vi "3_Extract Numbers_solution.vi"(11 "String":string="yi 2 -3 4.0 5.5") -> (3 "Result: Extracted Numbers":dbl[](array[numeric]) format="%#.6g")   [LabVIEW 2014]
panel:
  # "Extract Numbers from string and display in an array.\nThis picture is an example"
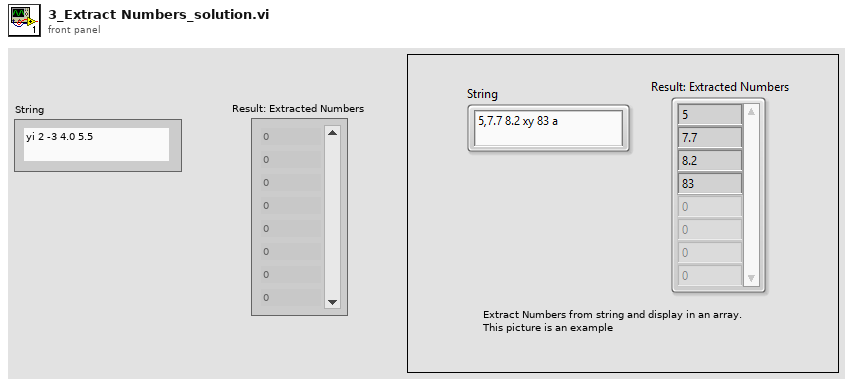
[diagram p1: front panel]
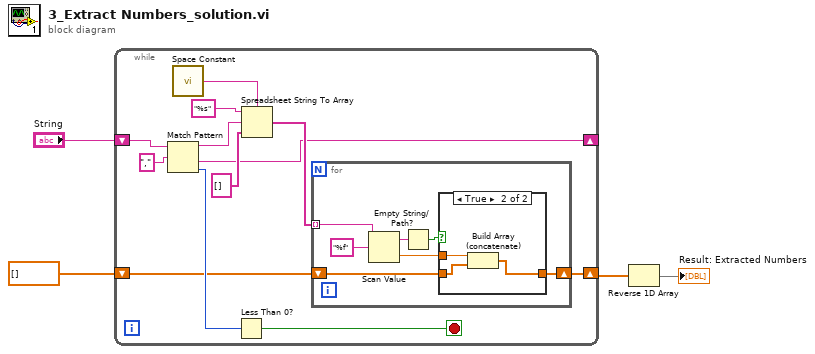
[diagram p0: block diagram]
diagram:
  n1 = while {
    shift-right: [w6] -> _
    shift-left: "String" -> [w16]
    shift-right: [w9] -> w2
    shift-left: dbl[] [] -> [w10]
    stop <- w13 stop-if-true
    n2 = Match Pattern(string=w16, regular expression=",") -> (before substring=w7:string, after substring=w6:string, offset past match=w14:i32)  [unwired: 1 in, 1 out]
    n3 = call <vilib>:"Space Constant.vi"() -> ("String"=w5:string)
    n4 = Less Than 0?(x=w14) -> (x < 0?=w13:bool)
    n5 = Spreadsheet String To Array(delimiter (Tab)=w5, format string="%s", spreadsheet string=w7, array type (2D Dbl)=string[] []) -> (array=w8:string[])
    n6 = for {
      shift-right: [w17] -> w9
      shift-left: w10 -> [w18]
      tunnel: w8 -> [w23] mode=indexing
      n7 = Scan Value(string=w23, format string="%f") -> (output string=w20:string, value=w19:dbl)  [unwired: 1 in]
      n8 = Empty String/Path?(string/path=w20) -> (empty?=w21:bool)
      n9 = case shown="True" w21 {
        tunnel: w19 -> [_ w27]
        tunnel: w18 -> [w24 w26]
        tunnel: [w24 w25] -> w17
        frame False {
        }
        frame True {
          n10 = Build Array (concatenate)(w27, w26) -> (w25:dbl[])
        }
      }
    }
  }
  n11 = Reverse 1D Array(array=w2) -> (reversed array=→"Result: Extracted Numbers":dbl[])
